vi "ProdaNG.Example.GetTestSteps.vi"() -> ()   [LabVIEW 2016]
uses:
  Controls/ProdaNG.Identification.ctl
  Controls/ProdaNG.TestStep.ctl
  Controls/ProdaNG.ProcessStep.ctl
  Controls/ProdaNG.Process.ctl
  Controls/ProdaNG.ProcessStepParam.ctl
  <vilib>/Utility/miscctls.llb/LVRowAndColumnUnsignedTypeDef.ctl
panel:
  in  "ResultStatus":i32(listbox)
  out "Identification":T1
  in  "ButtonUpdate":bool
  in  "ButtonRead":bool
  in  "Results":i32(listbox)
  out "ProcStepParams":T2[](array[typedef])
  out "Process":T3
  out "ProcStep":T4[](array[typedef])
  out "TestSteps":T5[](array[typedef])
  in  "Product Serial Number":string="123456789"
  out "ID":T6
  in  "Systems":u16(ring)=24 items=["AS110_TWIN", "AS120_TWIN", "AS130_TWIN", "AS140_TWIN", "AS220_TWIN", "AS230_TWIN", "AS240_TWIN", "AS310_TWIN", "AS320_TWIN", "AS330_TWIN", "AS340_TWIN", "AS410_TWIN", "AS420_TWIN", "AS430_TWIN", "AS510_TWIN", "AS520_TWIN", "AS530_TWIN", "AS610_TWIN", "AS620_TWIN", "AS710_TWIN", "AS_004_BSV", "AS_006.01_BSV_LASER", "AS_NT120_AMT", "AS_NT120_D_AMT", "AS_NT120_S_AMT", "AS_NT130B_AMT", "AS_NT130C_AMT", "AS_NT130D_AMT", "AS_NT130E_AMT", "AS_NT130_AMT", "AS_NT135_AMT", "AS_NT15_AMT", "AS_NT40_AMT", "AS_NT40_G_AMT", "AS_NT40_S_AMT", "AS_NT45_AMT", "AS_NT50_AMT", "NT60_FETT", "NT_110", "Q-CHECK_AMT", "TB_005.01.A_BSV", "TB_005.01.B_BSV", "TB_NT115.1_AMT", "TB_NT115.2_AMT", "TB_NT30_AMT", "TB_RANGE", "TB_RANGE_D", "TB_RANGE_RFID", "TB_TWIN", "VPGATES30.A", "VPGATES30.B", "unknown"]
  in  "Wabco Number":u16(ring)=191 items=["1111111111", "2222222222", "3333333333", "4154061010", "4154061020", "4154061050", "4154061060", "4154064020", "4154064040", "4154064050", "4154064060", "4154066001", "4154066031", "4154069362", "4154069432", "4213520020", "4213520030", "4213520995", "4213529995", "4213530070", "4213530077", "4213534000", "4213534010", "4213534020", "4213534030", "4213534040", "4213536000", "4213536010", "4213536020", "4213539991", "4213539993", "4213539994", "4213539995", "4213539997", "4213539999", "4213705342", "4430203001", "4430203021", "4430203041", "4430203051", "4461570050", "4463530000", "8840119999", "8840492280", "8840494770", "8840494790", "8840497570", "8840990060", "9140300130", "9549999910", "9640050050", "9640050060", "9640050070", "9640050080", "9999999404", "9999999405", "unknown"]
  in  "Connection string":string="lcptb/lcptb@PRODA_WPL"
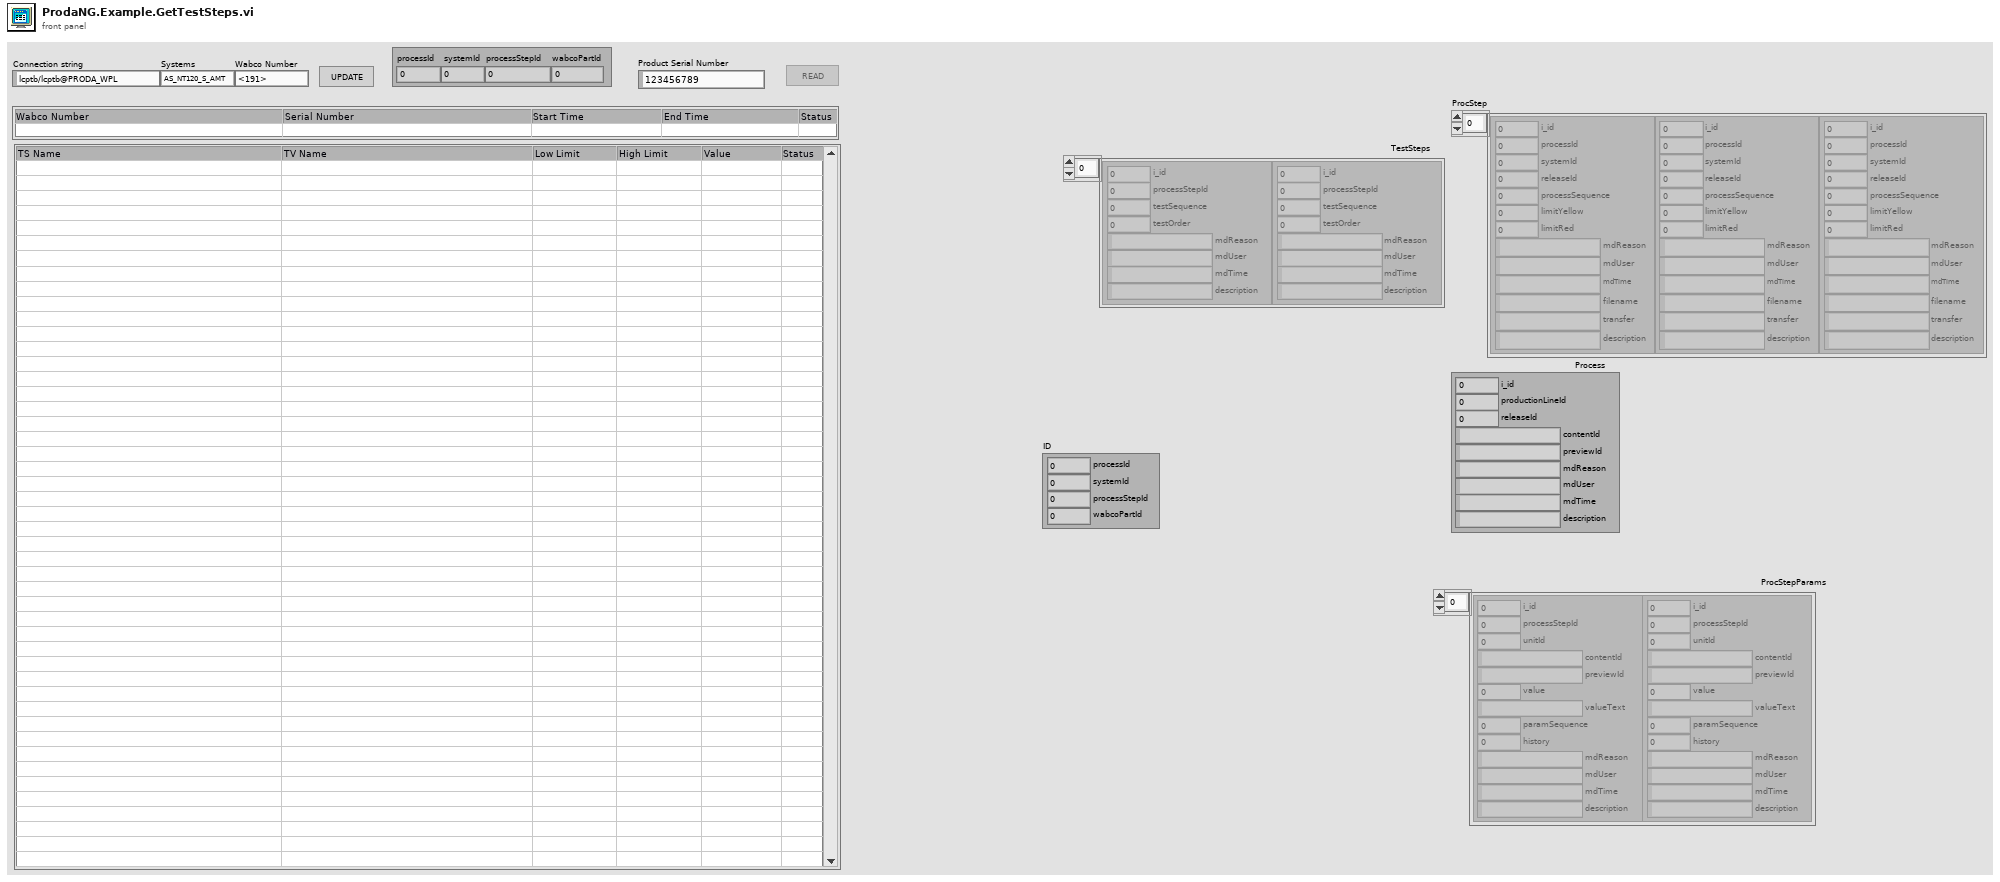
[diagram p1: front panel]
types:
  T1 = cluster{"processId":i32, "systemId":i32, "processStepId":i32, "wabcoPartId":i32}
  T2 = typedef "ProdaNG.ProcessStepParam.ctl" = cluster{"i_id":i32, "processStepId":i32, "unitId":i32, "contentId":string, "previewId":string, "value":dbl, "valueText":string, "paramSequence":i32, "history":i32, "mdReason":string, "mdUser":string, "mdTime":string, "description":string}
  T3 = typedef "ProdaNG.Process.ctl" = cluster{"i_id":i32, "productionLineId":i32, "releaseId":i32, "contentId":string, "previewId":string, "mdReason":string, "mdUser":string, "mdTime":string, "description":string}
  T4 = typedef "ProdaNG.ProcessStep.ctl" = cluster{"i_id":i32, "processId":i32, "systemId":i32, "releaseId":i32, "processSequence":i32, "limitYellow":dbl, "limitRed":dbl, "mdReason":string, "mdUser":string, "mdTime":string, "filename":string, "transfer":string, "description":string}
  T5 = typedef "ProdaNG.TestStep.ctl" = cluster{"i_id":i32, "processStepId":i32, "testSequence":i32, "testOrder":i32, "mdReason":string, "mdUser":string, "mdTime":string, "description":string}
  T6 = typedef "ProdaNG.Identification.ctl" = cluster{"processId":i32, "systemId":i32, "processStepId":i32, "wabcoPartId":i32}
  T7 = enum8{"Enabled", "Disabled", "Disabled and Grayed Out"}
  T8 = typedef "LVRowAndColumnUnsignedTypeDef.ctl" = cluster{"Row":u32, "Column":u32}
  T9 = typedef "ProdaNG.WabcoPart.ctl" = cluster{"i_id":i32, "workCenterId":i32, "contentId":string, "previewId":string, "mdReason":string, "mdUser":string, "mdTime":string, "productName":string, "wabcoNumber":string}
  T10 = typedef "ProdaNG.System.ctl" = cluster{"i_id":i32, "description":string}
  T11 = typedef "ProdaNG.Product.ctl" = cluster{"c_id":string, "wabcoPartId":i32, "serialNumber":string, "comment":string, "individual":i32, "crProcessStepId":i32, "mdProcessStepId":i32, "crTime":string, "mdTime":string}
  T12 = typedef "ProdaNG.ProcessResult.ctl" = cluster{"c_id":string, "productId":string, "processId":i32, "statusId":i32, "startTime":string, "endTime":string}
  T13 = typedef "ProdaNG.ProcessStepResult.ctl" = cluster{"c_id":string, "processResultId":string, "processStepId":i32, "statusId":i32, "operatorId":i32, "startTime":string, "endTime":string}
  T14 = typedef "ProdaNG.TestStepResult.ctl" = cluster{"c_id":string, "processStepResultId":string, "testStepId":i32, "statusId":i32}
  T15 = typedef "ProdaNG.TestValue.ctl" = cluster{"i_id":i32, "testStepId":i32, "releaseId":i32, "unitId":i32, "contentId":string, "previewId":string, "maximum":dbl, "minimum":dbl, "valueText":string, "testValueSequence":i32, "history":i32, "mdReason":string, "mdUser":string, "mdTime":string, "description":string}
  T16 = typedef "ProdaNG.TestValueResult.ctl" = cluster{"c_id":string, "testStepResultId":string, "testValueId":i32, "result":dbl, "statusId":i32, "contentId":string}
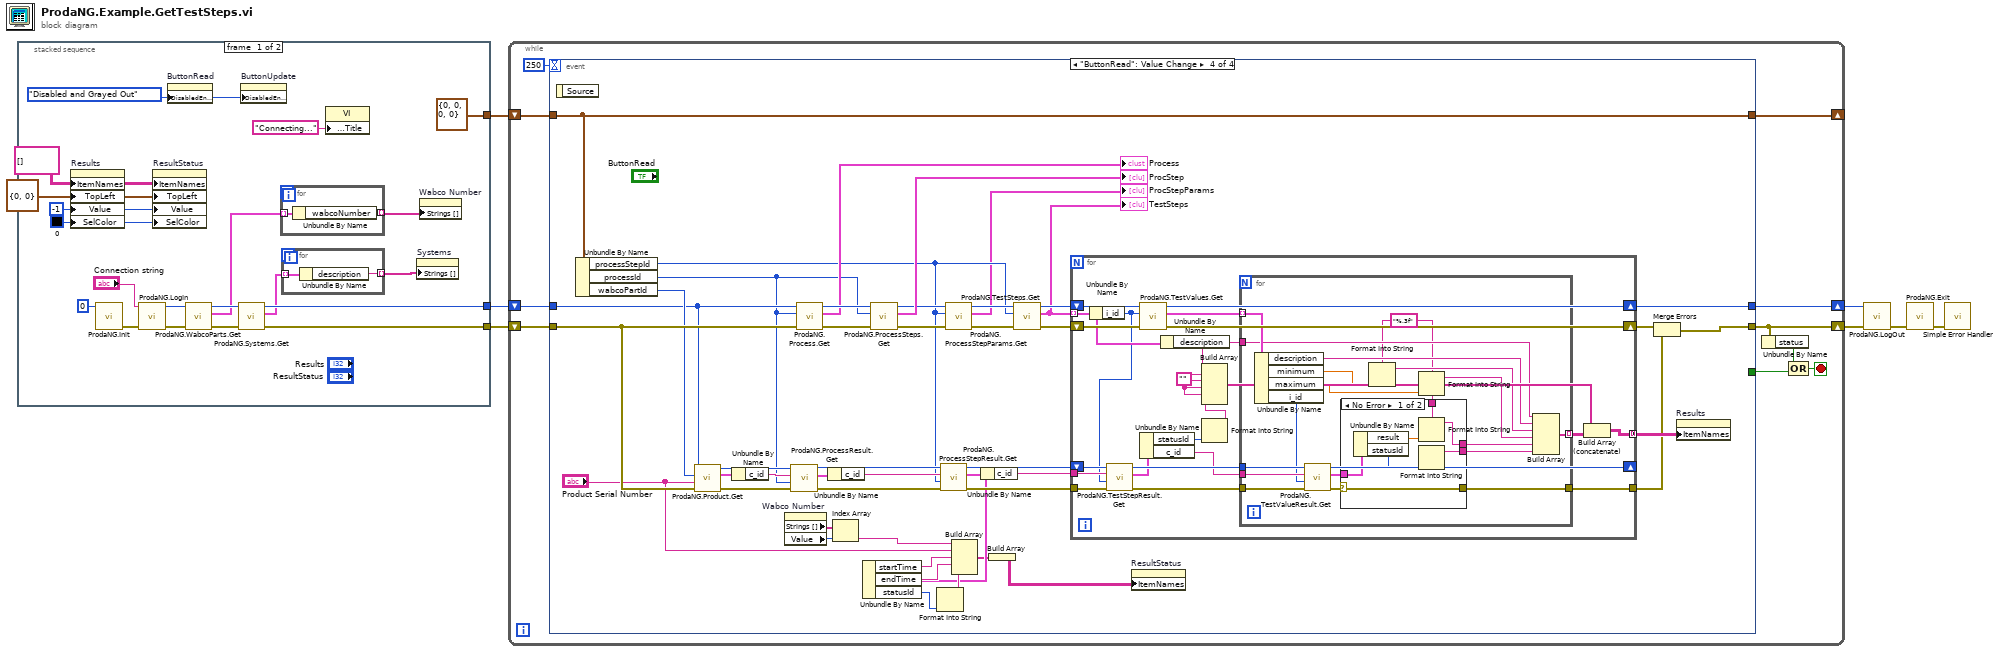
[diagram p0: block diagram]
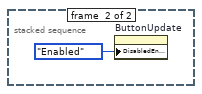
[diagram p2: hidden frame]
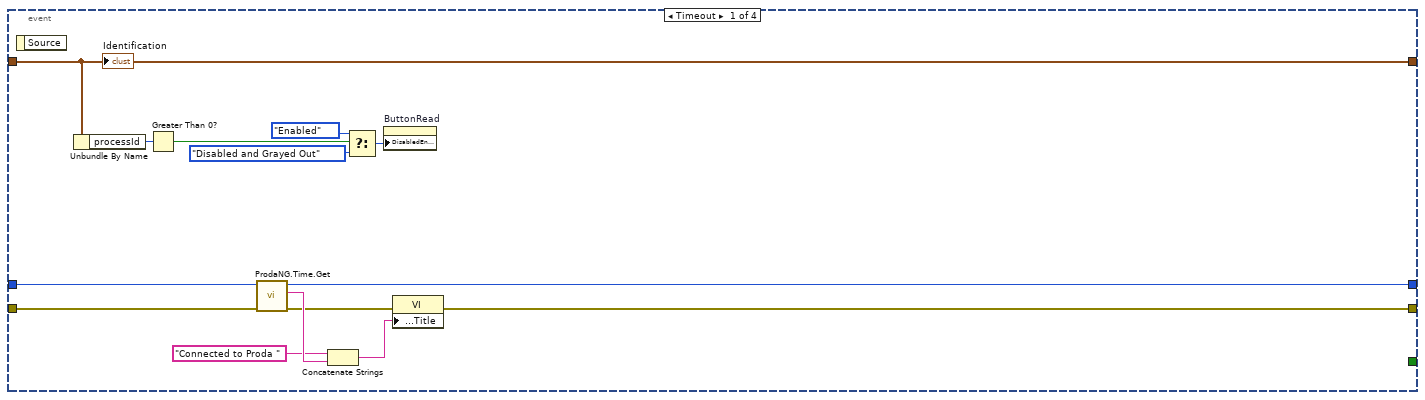
[diagram p3: hidden frame]
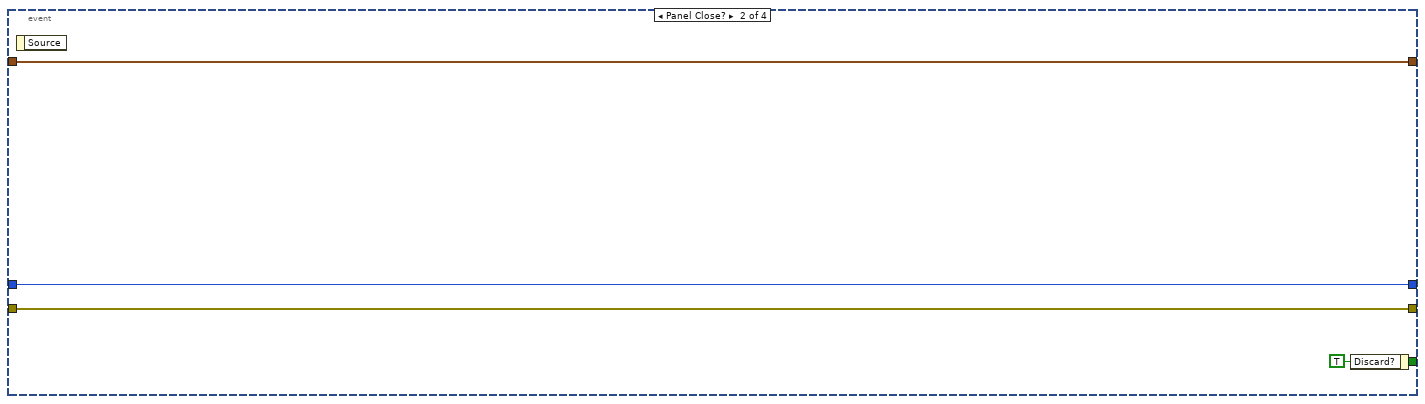
[diagram p4: hidden frame]
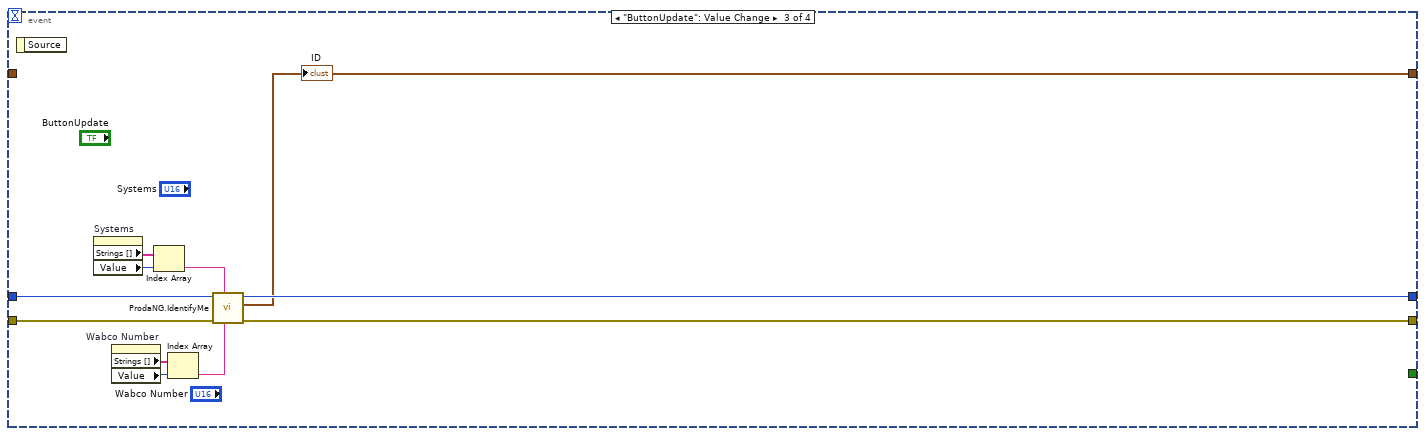
[diagram p5: hidden frame]
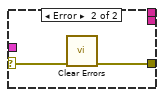
[diagram p6: hidden frame]
diagram:
  n1 = stacked-sequence {
    tunnel: [w22 _] -> w4
    tunnel: [w15 _] -> w3
    tunnel: [T6 {"processId"=0, "systemId"=0, "processStepId"=0, "wabcoPartId"=0} ("Identification") _] -> w2
    frame #0 {
      w13 = T7."Disabled and Grayed Out" ("Disabled")
      w9 = u32 0
      w8 = -1 ("Results")
      w10 = T8 {"Row"=0, "Column"=0} ("Top Left Visible Cell")
      w11 = string[][] [] ("Item Names")
      n2 = property on="Results" class="MCListbox (strict)"("ItemNames"=w11, "TopLeft"=w10, "Value"=w8, "SelColor"=w9) -> ()  [unwired: 2 in, 2 out]
      n3 = call "ProdaNG.Init.vi"("numContexts (0: unlimited)"=0 ("numContexts")) -> ("error out"=w27:errorcluster)  [unwired: 10 in]
      n4 = call "ProdaNG.LogIn.vi"("error in"=w27, "ConnectionString"="Connection string") -> ("error out"=w20:errorcluster, "dbHandle"=w24:i32)  [unwired: 7 in, 1 out]
      n5 = property on="ResultStatus" class="MCListbox (strict)"("ItemNames"=w11, "TopLeft"=w10, "Value"=w8, "SelColor"=w9) -> ()  [unwired: 2 in, 2 out]
      n6 = property on="ButtonRead" class="Bool"("DisabledEnum"=w13) -> ()  [unwired: 2 in, 2 out]
      n7 = call "ProdaNG.WabcoParts.Get.vi"("error in (no error)"=w20, "dbHandleIn"=w24) -> ("error out"=w21:errorcluster, "WabcoParts"=w17:T9[], "dbHandle"=w23:i32)  [unwired: 7 in]
      n8 = call "ProdaNG.Systems.Get.vi"("error in (no error)"=w21, "dbHandleIn"=w23) -> ("error out"=w15:errorcluster, "Systems"=w19:T10[], "dbHandle"=w22:i32)  [unwired: 7 in]
      n9 = property on="ButtonUpdate" class="Bool"("DisabledEnum"=w13) -> ()  [unwired: 2 in, 2 out]
      n10 = for {
        tunnel: w17 -> [w29] mode=indexing
        tunnel: [w28] -> w16 mode=indexing
        n11 = Unbundle By Name(w29) -> ("wabcoNumber"=w28:string)
      }
      n12 = for {
        tunnel: w19 -> [w31] mode=indexing
        tunnel: [w30] -> w18 mode=indexing
        n13 = Unbundle By Name(w31) -> ("description"=w30:string)
      }
      n14 = property class="VI"("Front Panel.Title"="Connecting..." ("Front Panel Window:Title")) -> ()  [unwired: 2 in, 2 out]
      n15 = property on="Systems" class="Ring (strict)"("Strings []"=w18) -> ()  [unwired: 2 in, 2 out]
      n16 = property on="Wabco Number" class="Ring (strict)"("Strings []"=w16) -> ()  [unwired: 2 in, 2 out]
    }
    frame #1 {
      n17 = property on="ButtonUpdate" class="Bool"("DisabledEnum"=T7."Enabled" ("Disabled")) -> ()  [unwired: 2 in, 2 out]
    }
  }
  n18 = while {
    shift-right: [w36] -> w5
    shift-left: w3 -> [w41]
    shift-right: [w42] -> w6
    shift-left: w4 -> [w40]
    shift-right: [w38] -> _
    shift-left: w2 -> [w37]
    stop <- w33 stop-if-true
    n19 = event shown="[3] \"ButtonRead\": Value Change" {
      selector: _ -> [_ _ _ _]
      dyn-events: _ -> [_ _ _ _]
      timeout: 250 -> [_ _ _ _]
      tunnel: [w54 w57 w68 w105] -> w42
      tunnel: w41 -> [w55 w58 w70 w103]
      tunnel: w40 -> [w56 w57 w71 w97]
      tunnel: [w43 w58 w69 w89] -> w36
      tunnel: [w48 w60 w67 w83] -> w38
      tunnel: w37 -> [w48 w60 _ w83]
      tunnel: [_ w59 _ _] -> w35
      event Timeout {
        n20 = event-data() -> ()  [unwired: 1 in, 1 out]
        n21 = Unbundle By Name(w48) -> ("processId"=w53:i32)
        n22 = Greater Than 0?(x=w53) -> (x > 0?=w52:bool)
        n23 = call "ProdaNG.Time.Get.vi"("error in"=w55, "dbHandleIn"=w56) -> ("error out"=w44:errorcluster, "timeStr"=w47:string, "dbHandle"=w54:i32)  [unwired: 5 in, 1 out]
        n24 = Concatenate Strings("Connected to Proda " ("string"), w47) -> (w46:string)
        n25 = Select(t=T7."Enabled" ("Disabled"), s=w52, f=T7."Disabled and Grayed Out" ("Disabled")) -> (s? t:f=w51:T7)
        n26 = property on="ButtonRead" class="Bool"("DisabledEnum"=w51) -> ()  [unwired: 2 in, 2 out]
        n27 = property class="VI"(error in=w44, "Front Panel.Title"=w46) -> (error out=w43:errorcluster)  [unwired: 1 in, 1 out]
        "Identification" <- w48
      }
      event Panel Close? {
        w59 = TRUE ("Discard?")
        n28 = event-data() -> ()  [unwired: 1 in, 1 out]
        n29 = event-data("Discard?"=w59) -> ()  [unwired: 1 in, 1 out]
      }
      event "ButtonUpdate": Value Change {
        n30 = event-data() -> ()  [unwired: 1 in, 1 out]
        n31 = property on="Systems" class="Ring (strict)"() -> ("Strings []"=w63:string[], "Value"=w62:u16)  [unwired: 2 in, 2 out]
        n32 = property on="Wabco Number" class="Ring (strict)"() -> ("Strings []"=w65:string[], "Value"=w66:u16)  [unwired: 2 in, 2 out]
        n33 = Index Array(array=w63, index=w62) -> (element=w61:string)
        n34 = Index Array(array=w65, index=w66) -> (element=w64:string)
        n35 = call "ProdaNG.IdentifyMe.vi"("wabcoNumber"=w64, "systemName"=w61, "error in"=w70, "dbHandleIn"=w71) -> ("error out"=w69:errorcluster, "Identification"=w67:T6, "dbHandle"=w68:i32)  [unwired: 5 in]
        "ID" <- w67
      }
      event "ButtonRead": Value Change {
        n36 = event-data() -> ()  [unwired: 1 in, 1 out]
        n37 = Unbundle By Name(w83) -> ("processStepId"=w92:i32, "processId"=w96:i32, "wabcoPartId"=w102:i32)
        n38 = call "ProdaNG.Product.Get.vi"("error in (no error)"=w103, "serialNumber"="Product Serial Number", "wabcoPartId"=w102, "dbHandle"=w97) -> ("error out"=w101:errorcluster, "Product"=w99:T11, "dbHandle out"=w98:i32)  [unwired: 4 in, 1 out]
        n39 = Unbundle By Name(w99) -> ("c_id"=w100:string)
        n40 = property on="Wabco Number" class="Ring (strict)"() -> ("Strings []"=w76:string[], "Value"=w77:u16)  [unwired: 2 in, 2 out]
        n41 = call "ProdaNG.ProcessResult.Get.vi"("error in (no error)"=w101, "processId"=w96, "productId"=w100, "dbHandle"=w98) -> ("error out"=w93:errorcluster, "ProcessResult"=w87:T12, "dbHandle out"=w94:i32)  [unwired: 4 in, 1 out]
        n42 = call "ProdaNG.Process.Get.vi"("error in (no error)"=w103, "processId"=w96, "dbHandleIn"=w97) -> ("error out"=w115:errorcluster, "Process"=→"Process":T3, "dbHandle"=w114:i32)  [unwired: 5 in, 1 out]
        n43 = Unbundle By Name(w87) -> ("c_id"=w95:string)
        n44 = Index Array(array=w76, index=w77) -> (element=w75:string)
        n45 = call "ProdaNG.ProcessSteps.Get.vi"("error in (no error)"=w115, "processId"=w96, "dbHandleIn"=w114) -> ("error out"=w111:errorcluster, "ProcSteps"=→"ProcStep":T4[], "dbHandle"=w112:i32)  [unwired: 6 in]
        n46 = call "ProdaNG.ProcessStepResult.Get.vi"("error in (no error)"=w93, "processStepId"=w92, "processResultId"=w95, "dbHandle"=w94) -> ("error out"=w91:errorcluster, "ProcessStepResult"=w74:T13, "dbHandle out"=w90:i32)  [unwired: 4 in, 1 out]
        n47 = Unbundle By Name(w74) -> ("startTime"=w81:string, "endTime"=w80:string, "statusId"=w79:i32)
        n48 = Format Into String(w79) -> (resulting string=w78:string)  [unwired: 3 in, 1 out]
        n49 = call "ProdaNG.ProcessStepParams.Get.vi"("error in (no error)"=w111, "processStepId"=w92, "dbHandleIn"=w112) -> ("error out"=w110:errorcluster, "ProcStepParams"=→"ProcStepParams":T2[], "dbHandle"=w109:i32)  [unwired: 6 in]
        n50 = Build Array(w75, "Product Serial Number", w81, w80, w78) -> (w73:string[])
        n51 = Unbundle By Name(w74) -> ("c_id"=w88:string)
        n52 = Build Array(w73) -> (w72:string[][])
        n53 = call "ProdaNG.TestSteps.Get.vi"("error in (no error)"=w110, "processStepId"=w92, "dbHandleIn"=w109) -> ("error out"=w107:errorcluster, "TestSteps"=w106:T5[], "dbHandle"=w108:i32)  [unwired: 6 in]
        "TestSteps" <- w106
        n54 = for {
          tunnel: w106 -> [w129] mode=indexing
          shift-right: [w136] -> w105
          shift-left: w108 -> [w137]
          shift-right: [w135] -> w104
          shift-left: w107 -> [w138]
          shift-right: [w132] -> _
          shift-left: w90 -> [w134]
          tunnel: w88 -> [w133]
          tunnel: [w121] -> w86 mode=concatenating
          tunnel: w91 -> [w126]
          tunnel: [w128] -> w84
          w122 = ""
          n55 = Unbundle By Name(w129) -> ("i_id"=w118:i32)
          n56 = call "ProdaNG.TestStepResult.Get.vi"("error in (no error)"=w126, "testStepId"=w118, "processStepResulttId"=w133, "dbHandle"=w134) -> ("error out"=w127:errorcluster, "TestStepResult"=w117:T14, "dbHandle out"=w132:i32)  [unwired: 4 in, 1 out]
          n57 = call "ProdaNG.TestValues.Get.vi"("error in (no error)"=w138, "testStepId"=w118, "dbHandleIn"=w137) -> ("error out"=w135:errorcluster, "TestStepValues"=w131:T15[], "dbHandle"=w136:i32)  [unwired: 6 in]
          n58 = Unbundle By Name(w117) -> ("statusId"=w124:i32, "c_id"=w119:string)
          n59 = Unbundle By Name(w129) -> ("description"=w125:string)
          n60 = Format Into String(w124) -> (resulting string=w123:string)  [unwired: 3 in, 1 out]
          n61 = Build Array(w125, w122, w122, w122, w122, w123) -> (w120:string[])
          n62 = for {
            tunnel: w119 -> [w156]
            tunnel: w132 -> [w155]
            tunnel: w127 -> [w154]
            tunnel: w131 -> [w153] mode=indexing
            tunnel: [w149] -> w130 mode=indexing
            tunnel: w125 -> [w146]
            tunnel: [w144] -> w128
            w139 = "%.3f" ("format string")
            n63 = Unbundle By Name(w153) -> ("description"=w147:string, "minimum"=w143:dbl, "maximum"=w140:dbl, "i_id"=w152:i32)
            n64 = call "ProdaNG.TestValueResult.Get.vi"("error in (no error)"=w154, "testValueId"=w152, "testStepResultId"=w156, "dbHandle"=w155) -> ("error out"=w145:errorcluster, "TestValueResult"=w151:T16)  [unwired: 5 in, 1 out]
            n65 = case shown="No Error" w145 {
              selector: w145 -> [w158 w165]
              tunnel: w151 -> [w163 _]
              tunnel: [w161 _] -> w150
              tunnel: [w160 _] -> w148
              tunnel: [w158 w164] -> w144
              tunnel: w139 -> [w157 _]
              frame No Error {
                n66 = Unbundle By Name(w163) -> ("result"=w162:dbl, "statusId"=w159:i32)
                n67 = Format Into String(format string=w157, w162) -> (resulting string=w160:string)  [unwired: 2 in, 1 out]
                n68 = Format Into String(w159) -> (resulting string=w161:string)  [unwired: 3 in, 1 out]
              }
              frame Error {
                n69 = call <vilib>:"Clear Errors.vi"("error in (no error)"=w165) -> ("error out"=w164:errorcluster)  [unwired: 5 in, 1 out]
              }
            }
            n70 = Format Into String(format string=w139, w143) -> (resulting string=w141:string)  [unwired: 2 in, 1 out]
            n71 = Format Into String(format string=w139, w140) -> (resulting string=w142:string)  [unwired: 2 in, 1 out]
            n72 = Build Array(w146, w147, w141, w142, w148, w150) -> (w149:string[])
          }
          n73 = Build Array (concatenate)(w120, w130) -> (w121:string[][])
        }
        n74 = property on="ResultStatus" class="MCListbox (strict)"("ItemNames"=w72) -> ()  [unwired: 2 in, 2 out]
        n75 = Merge Errors(w104, w84) -> (w89:errorcluster)
        n76 = property on="Results" class="MCListbox (strict)"("ItemNames"=w86) -> ()  [unwired: 2 in, 2 out]
      }
    }
    n77 = Unbundle By Name(w36) -> ("status"=w34:bool)
    n78 = Compound Arithmetic op=OR(w34, w35) -> (w33:bool)
  }
  n79 = call "ProdaNG.LogOut.vi"("error in"=w5, "dbHandleIn"=w6) -> ("error out"=w7:errorcluster)  [unwired: 9 in]
  n80 = call "ProdaNG.Exit.vi"("error in (no error)"=w7) -> ("error out"=w1:errorcluster)  [unwired: 10 in]
  n81 = call <vilib>:"Simple Error Handler.vi"("error in (no error)"=w1) -> ()  [unwired: 4 in, 5 out]
